vi "GetCurrentPosition.vi"(8 "error in (no error)":errorcluster, 11 "Serial Controller in":refnum<class "Serial Controller.lvclass">) -> (0 "error out":errorcluster, 1 "PositionBundle":cluster{"X":dbl, "Y":dbl, "Z":dbl, "Depth":dbl}, 2 "Position":dbl[](array[numeric]), 3 "Serial Controller out":refnum<class "Serial Controller.lvclass">)   [LabVIEW 2014, in "Serial Controller.lvclass"]
uses:
  Serial Controller.lvclass
  Serial Controller.lvclass/Serial Controller.ctl
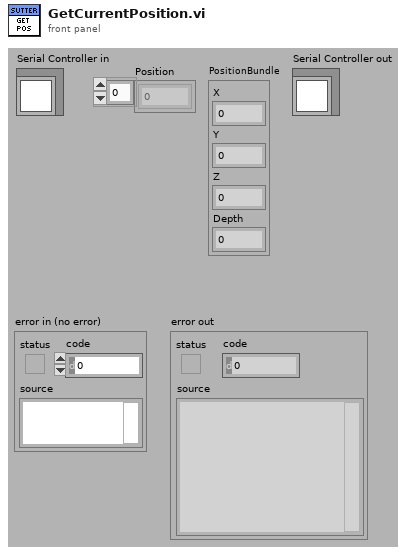
[diagram p1: front panel]
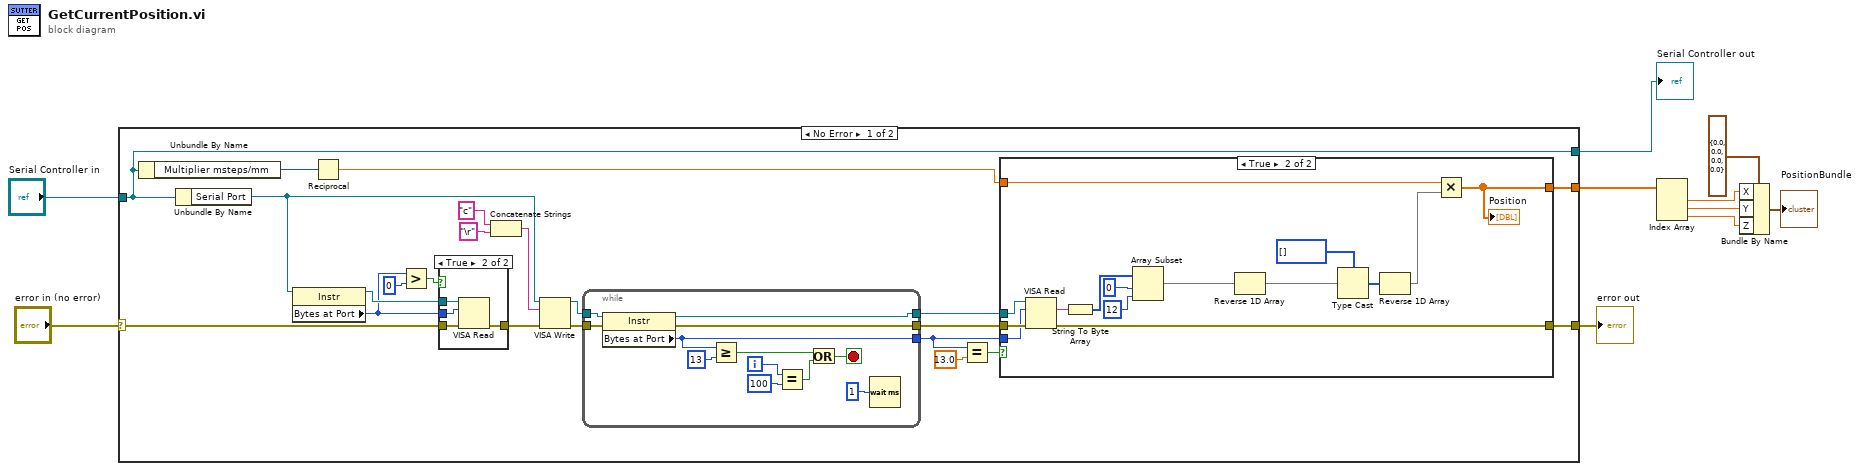
[diagram p0: block diagram]
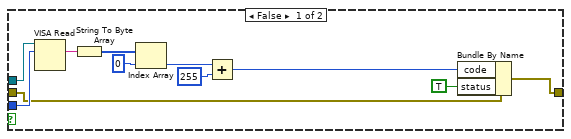
[diagram p2: hidden frame]
diagram:
  n1 = case shown="No Error" "error in (no error)" {
    selector: "error in (no error)" -> [w20 w76]
    tunnel: [w18 w76] -> w3
    tunnel: [w26 w75] -> w9
    tunnel: "Serial Controller in" -> [w26 w75]
    tunnel: [w32 _] -> w7
    frame No Error {
      n2 = Unbundle By Name(w26) -> ("Multiplier msteps/mm"=w11:i16)
      n3 = Unbundle By Name(w26) -> ("Serial Port"=w24:refnum<visa-resource-name>)
      n4 = property class="Instr"(reference=w24) -> (reference out=w22:refnum<visa-resource-name>, "Bytes at Port"=w21:u32)  [unwired: 1 in, 1 out]
      n5 = Reciprocal(x=w11) -> (1/x=w12:dbl)
      n6 = Greater?(x=w21, y=u32 0) -> (0:w25:bool)
      n7 = case shown="True" w25 {
        tunnel: w22 -> [_ w62]
        tunnel: w21 -> [_ w61]
        tunnel: w20 -> [_ w60]
        tunnel: [_ w59] -> w19
        frame False {
        }
        frame True {
          n8 = VISA Read(VISA resource name=w62, byte count=w61, error in (no error)=w60) -> (error out=w59:errorcluster)  [unwired: 3 out]
        }
      }
      n9 = Concatenate Strings("c" ("string"), "\r" ("write buffer")) -> (w28:string)
      n10 = VISA Write(VISA resource name=w24, write buffer=w28, error in (no error)=w19) -> (VISA resource name out=w31:refnum<visa-resource-name>, error out=w27:errorcluster)  [unwired: 1 out]
      n11 = while {
        tunnel: w31 -> [w74]
        tunnel: w27 -> [w73]
        tunnel: [w72] -> w13
        tunnel: [w70] -> w14
        tunnel: [w63] -> w16
        i -> [w66]
        stop <- w67 stop-if-true
        n12 = property class="Instr"(reference=w74, error in=w73) -> (reference out=w72:refnum<visa-resource-name>, error out=w70:errorcluster, "Bytes at Port"=w63:u32)
        n13 = Greater Or Equal?(x=w63, y=u32 13) -> (x >= y?=w68:bool)
        n14 = Equal?(x=w66, y=100) -> (x = y?=w64:bool)
        n15 = Or(x=w68, y=w64) -> (x .or. y?=w67:bool)
        n16 = Wait (ms)(milliseconds to wait=u32 1) -> ()  [unwired: 1 out]
      }
      n17 = Equal?(x=w16, y=13.0) -> (x = y?=w15:bool)
      n18 = case shown="True" w15 {
        tunnel: w12 -> [_ w50]
        tunnel: [_ w49] -> w32
        tunnel: w13 -> [w43 w48]
        tunnel: w14 -> [w40 w46]
        tunnel: [w34 w45] -> w18
        tunnel: w16 -> [w42 w44]
        frame False {
          n19 = VISA Read(VISA resource name=w43, byte count=w42) -> (read buffer=w41:string)  [unwired: 1 in, 3 out]
          n20 = String To Byte Array(string=w41) -> (unsigned byte array=w39:u8[])
          n21 = Index Array(array=w39, index=0) -> (element=w37:u8)
          n22 = Add(x=w37, y=u8 255) -> (x+y=w35:u8)
          n23 = Bundle By Name(cluster=w40, "code"=w35, "status"=TRUE) -> (w34:errorcluster)
        }
        frame True {
          n24 = VISA Read(VISA resource name=w48, byte count=w44, error in (no error)=w46) -> (read buffer=w47:string, error out=w45:errorcluster)  [unwired: 2 out]
          n25 = String To Byte Array(string=w47) -> (unsigned byte array=w58:u8[])
          n26 = Array Subset(array=w58, index=0, length=12) -> (w54:u8[])
          n27 = Reverse 1D Array(array=w54) -> (reversed array=w53:u8[])
          n28 = Type Cast(type=i32[] [], x=w53) -> (*(type *) &x=w52:i32[])
          n29 = Reverse 1D Array(array=w52) -> (reversed array=w51:i32[])
          n30 = Multiply(x=w50, y=w51) -> (x*y=w49:dbl[])
          "Position" <- w49
        }
      }
    }
    frame Error {
    }
  }
  "error out" <- w3
  "Serial Controller out" <- w9
  n31 = Index Array(array=w7) -> (element #1=w6:dbl, element #2=w5:dbl, element #3=w4:dbl)  [unwired: 3 in]
  n32 = Bundle By Name(cluster=cluster{"X":dbl, "Y":dbl, "Z":dbl, "Depth":dbl} {"X"=0.0, "Y"=0.0, "Z"=0.0, "Depth"=0.0} ("Cluster"), "X"=w6, "Y"=w5, "Z"=w4) -> (→"PositionBundle":cluster{"X":dbl, "Y":dbl, "Z":dbl, "Depth":dbl})
